vi "Perform Action.vi"(8 "error in":errorcluster, 10 "Input":variant, 11 "Virt Instrument Base in":refnum<class "Virt EL Measure Power DC CFG.lvclass">) -> (0 "error out":errorcluster, 2 "Output":variant, 3 "Virt Instrument Base out":refnum<class "Virt EL Measure Power DC CFG.lvclass">)   [LabVIEW 2023, in "Virt EL Measure Power DC CFG.lvclass"]
uses:
  Virt EL Measure Power DC CFG.lvclass
  Virt EL Measure Power DC CFG.lvclass/Virt EL Measure Power DC CFG.ctl
  Virt Instr Base/Virt Instr Base.lvclass
  5cce63ce-16b9-40b0-8e7d-0c2da8a6f844.vi
  SCPI PE Input.ctl
  Virt Instr Host/Virt Instr Local.lvclass
  D:/git/HAL/HAL GOOP4/Virt Instr Host/Virt Instr Local.lvclass
  D:/git/HAL/HAL GOOP4/Virt Instr Base/Virt Instr Base.lvclass
  D:/git/HAL/HAL GOOP4/Devices/Eletronic Load 9080/Configurations/Virtual Instruments/Virt EL Measure Power/Virt EL Measure Power DC CFG.lvclass
  Instrument/Instrument.lvclass
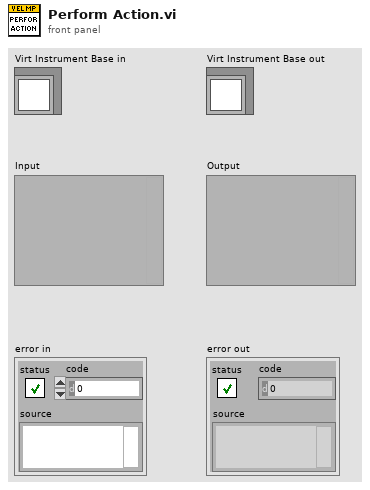
[diagram p1: front panel]
types:
  T1 = typedef "SCPI PE Input.ctl" = cluster{"Action":enum16{"Write", "Query"}, "SCPI":string}
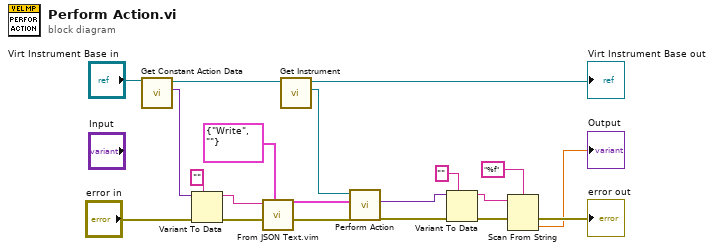
[diagram p0: block diagram]
diagram:
  n1 = call "Get Constant Action Data.vi"("Virt Instr Base in"="Virt Instrument Base in") -> ("Constant Action Data"=w11:variant, "Virt Instr Base out"=w7:refnum<class "Virt EL Measure Power DC CFG.lvclass">)  [unwired: 9 in]
  n2 = Variant To Data(error in="error in", type="", Variant=w11) -> (data=w9:string, error out=w10:errorcluster)
  n3 = call "From JSON Text.vim"("Data Type and Default Value"=T1 {"Action"=enum."Write", "SCPI"=""} ("PE Input"), "error in (no error)"=w10, "JSON"=w9) -> ("error out"=w6:errorcluster, "Data out"=w4:T1)  [unwired: 7 in]
  n4 = call "Get Instrument.vi"("Virt Instr Base in"=w7) -> ("HAL GOOP4.lvlib:Instrument"=w5:refnum<class "Instrument.lvclass">, "Virt Instr Base out"=→"Virt Instrument Base out":refnum<class "Virt EL Measure Power DC CFG.lvclass">)  [unwired: 9 in]
  n5 = call "Perform Action.vi"("Error In"=w6, "Input"=w4, "reference in"=w5) -> ("Error Out"=w3:errorcluster, "Output"=w2:variant)  [unwired: 6 in, 1 out]
  n6 = Variant To Data(error in=w3, type="", Variant=w2) -> (data=w17:string, error out=w20:errorcluster)
  n7 = Scan From String(format string="%f", input string=w17, error in=w20) -> (error out=→"error out":errorcluster, output 1=→"Output":dbl)  [unwired: 2 in, 2 out]
